vi "Set settings chain.vi"(8 "error in (no error)":errorcluster, 9 "class names":string[](array[string]), 10 "settings":variant[](array[variant]), 11 "ServiceManagerLoader in":refnum<class "ServiceManagerLoader.lvclass">) -> (0 "error out":errorcluster, 3 "ServiceManagerLoader out":refnum<class "ServiceManagerLoader.lvclass">)   [LabVIEW 2012, in "ServiceManagerLoader.lvclass"]
uses:
  ServiceManagerLoader.lvclass
  <vilib>/Distrio/Murmex/Murmex/Murmex.lvclass
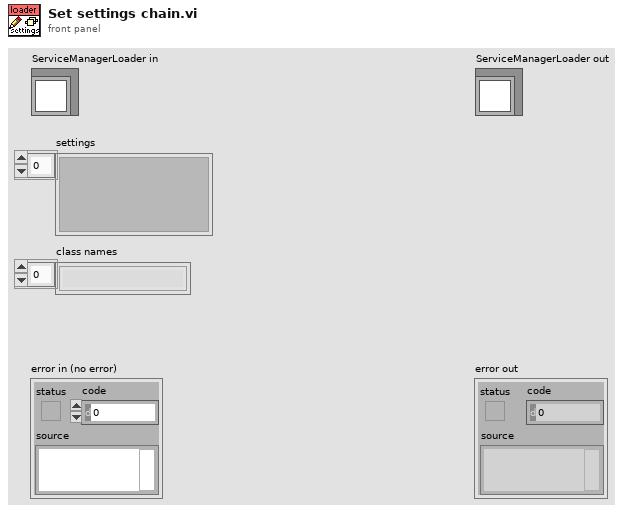
[diagram p1: front panel]
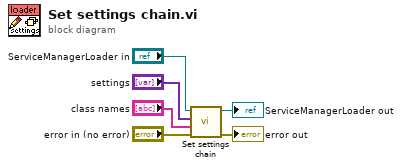
[diagram p0: block diagram]
diagram:
  n1 = call-parent "Set settings chain.vi"("error in (no error)"="error in (no error)", "class names"="class names", "settings"="settings", "Murmex in"="ServiceManagerLoader in") -> ("error out"=→"error out":errorcluster, "Murmex out"=→"ServiceManagerLoader out":refnum<class "ServiceManagerLoader.lvclass">)  [unwired: 6 in]
